vi "mk.vi"() -> ()   [LabVIEW 2016]
uses:
  <vilib>/Utility/file.llb/Write Delimited Spreadsheet (DBL).vi
panel:
  in  "Nombre (guardar como .txt)":path
  in  "cambio":bool
  out "campo":dbl
  in  "paso":dbl
  in  "final":dbl
  in  "inicio":dbl
  out "Lock_In":cluster{"array":dbl[], "array":dbl[]}(graph)
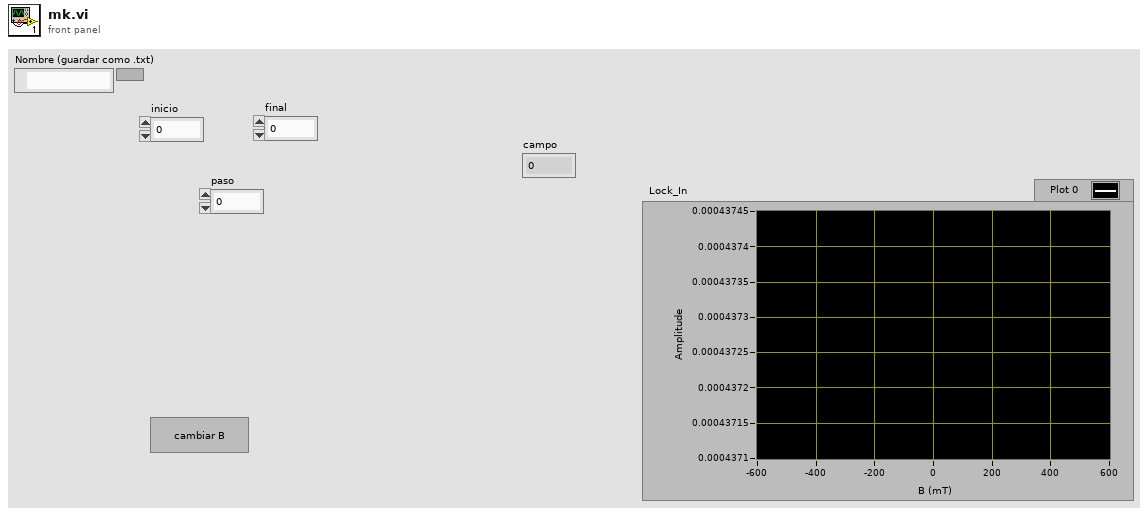
[diagram p1: front panel]
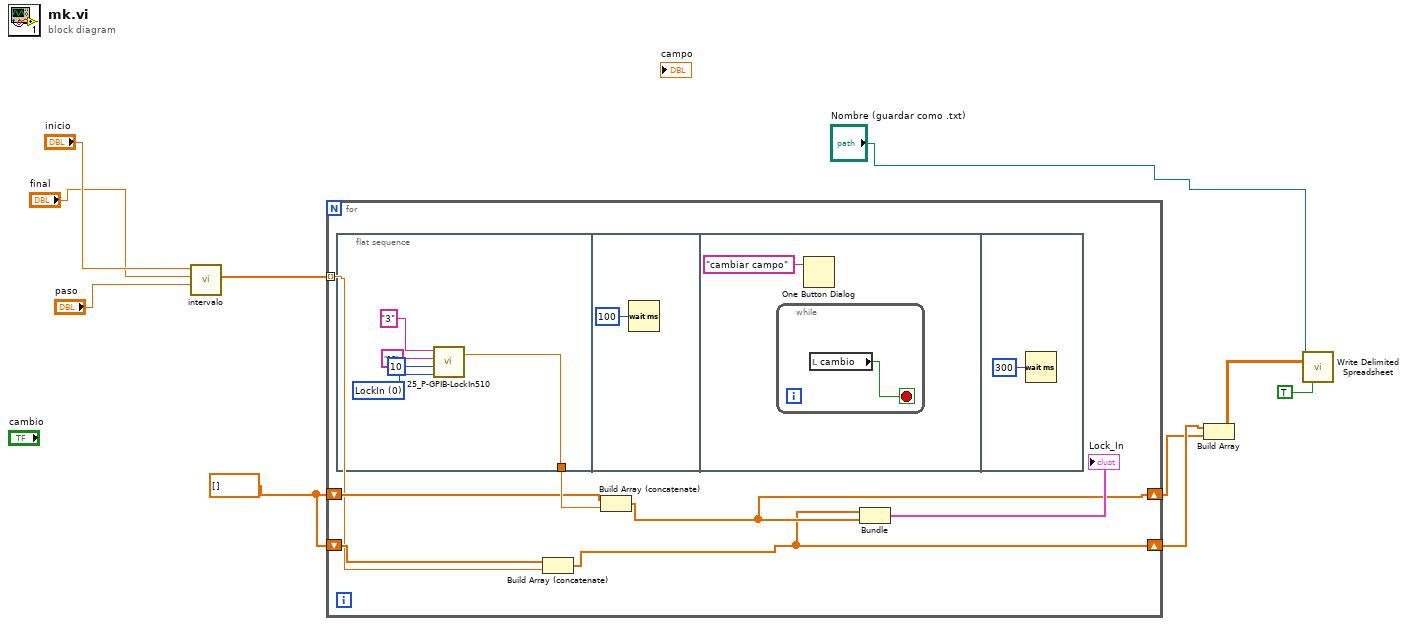
[diagram p0: block diagram]
diagram:
  w6 = dbl[] []
  n1 = call "intervalo.vi"("incremento"="paso", "fin"="final", "inicio"="inicio") -> ("Array"=w7:dbl[])  [unwired: 8 in]
  n2 = for {
    tunnel: w7 -> [w14] mode=indexing
    shift-right: [w12] -> w3
    shift-left: w6 -> [w16]
    shift-right: [w11] -> w4
    shift-left: w6 -> [w15]
    n3 = flat-sequence {
      tunnel: [w18] -> w17
      frame #0 {
        w19 = u16 0 items=["LockIn", "LockIn-DMM"] ("Tipo")
        n4 = call "25_P-GPIB-LockIn510.vi"("Tipo"=w19, "Lecturas"=10, "P-DMM"="16", "P-LockIn"="3") -> ("LockIn"=w18:dbl)  [unwired: 1 out]
      }
      frame #1 {
        n5 = Wait (ms)(milliseconds to wait=u32 100) -> ()  [unwired: 1 out]
      }
      frame #2 {
        n6 = while {
          stop <- w25 stop-if-true
          n7 = local read "cambio"() -> (w25:bool)
        }
        n8 = One Button Dialog(message="cambiar campo") -> ()  [unwired: 1 in, 1 out]
      }
      frame #3 {
        n9 = Wait (ms)(milliseconds to wait=u32 300) -> ()  [unwired: 1 out]
      }
    }
    n10 = Build Array (concatenate)(w15, w14) -> (w11:dbl[])
    n11 = Build Array (concatenate)(w16, w17) -> (w12:dbl[])
    n12 = Bundle(w11, w12) -> (→"Lock_In":cluster{dbl[], dbl[]})  [unwired: 1 in]
  }
  n13 = Build Array(w4, w3) -> (w2:dbl[][])
  n14 = call-poly <vilib>:"Write Delimited Spreadsheet.vi"("file path (dialog if empty)"="Nombre (guardar como .txt)", "2D data"=w2, "transpose? (no:F)"=TRUE) -> ()  [unwired: 11 in, 2 out]
